vi "MGCC_FntStaMach_Flagtoevent.vi"(6 "ABN_recover":bool, 7 "Flags":bool[](array[boolean]), 8 "error in":errorcluster, 9 "M_OFF":bool, 10 "Pre_state":string, 11 "ABN_state":string="State1:OFF") -> (1 "error out":errorcluster, 2 "Event":bool[](array[boolean]), 3 "Previous_state":string)   [LabVIEW 2016]
doc: "-----------------------------------------------------------------------------------------------------------------------\nCopyright <2019> <The University of Tennessee at Knoxville and the University of Tennessee Research Foundation>\nThis software is released under BSD-3 \nhttps://opensource.org/licenses/BSD-3-Clause \nAdditional license options available at https://utrf.tennessee.edu/industry/sample-agreements/\n-----------------------------------------------------------------------------------------------------------------------"
uses:
  <vilib>/imath/engines/lvmath/Plug In/_Char/NIMS_CH_character datatype.ctl
  <vilib>/Utility/error.llb/Error Cluster From Error Code.vi
  Unplanned islanding/Sub Vis/UnplanISD_Global.vi
  <vilib>/imath/engines/lvmath/Plug In/_Char/NIMS_CH_String to Character Array.vi
  <vilib>/imath/engines/lvmath2/RunTimeEngine/IndexRead/NIMS V(S).vi
  <instcachedir>/0/NIMS V(S)_0488751826AF41519A22953C041130DC.lvgen/NIMS V(S)_0488751826AF41519A22953C041130DC_003.vi
  <vilib>/imath/engines/lvmath2/RunTimeEngine/ErrorHandling/NIMS_Create Error From Enums.vi
  <vilib>/imathl/engines/lvmath/Functions/Error Handling/Create Error.vi
  <vilib>/imath/engines/lvmath2/RunTimeSupport/NIMS_Compare Aggregates.vi
  <instcachedir>/0/NIMS_Compare Aggregates_FA3EBEB3749E48D38A57888B5ABBF163.lvgen/NIMS_Compare Aggregates_FA3EBEB3749E48D38A57888B5ABBF163_000.vi
  <vilib>/imath/engines/lvmath2/RunTimeEngine/NodeEndStatement/NIMS_NodeEndStatement_Output.vi
  <instcachedir>/0/NIMS_NodeEndStatement_Output_53EC0D466D134D7ABD903AC30B43404B.lvgen/NIMS_NodeEndStatement_Output_53EC0D466D134D7ABD903AC30B43404B_013.vi
  <vilib>/imath/engines/lvmath/Plug In/_Char/NIMS_CH_Character RV to String.vi
  <instcachedir>/0/NIMS_NodeEndStatement_Output_53EC0D466D134D7ABD903AC30B43404B.lvgen/NIMS_NodeEndStatement_Output_53EC0D466D134D7ABD903AC30B43404B_008.vi
  <vilib>/imath/engines/lvmath2/RunTimeEngine/ErrorHandling/NIMS_Finalize Error.vi
  <vilib>/ErrorRing/Error Ring.xnode
panel:
  out "error out 2":errorcluster
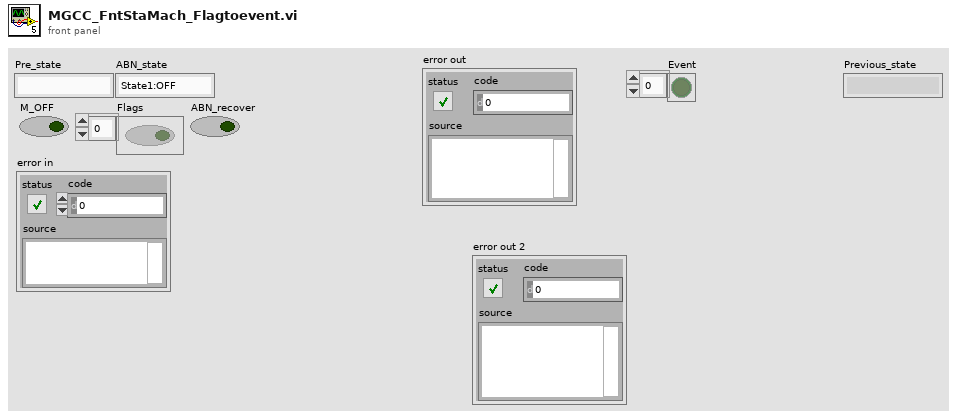
[diagram p1: front panel]
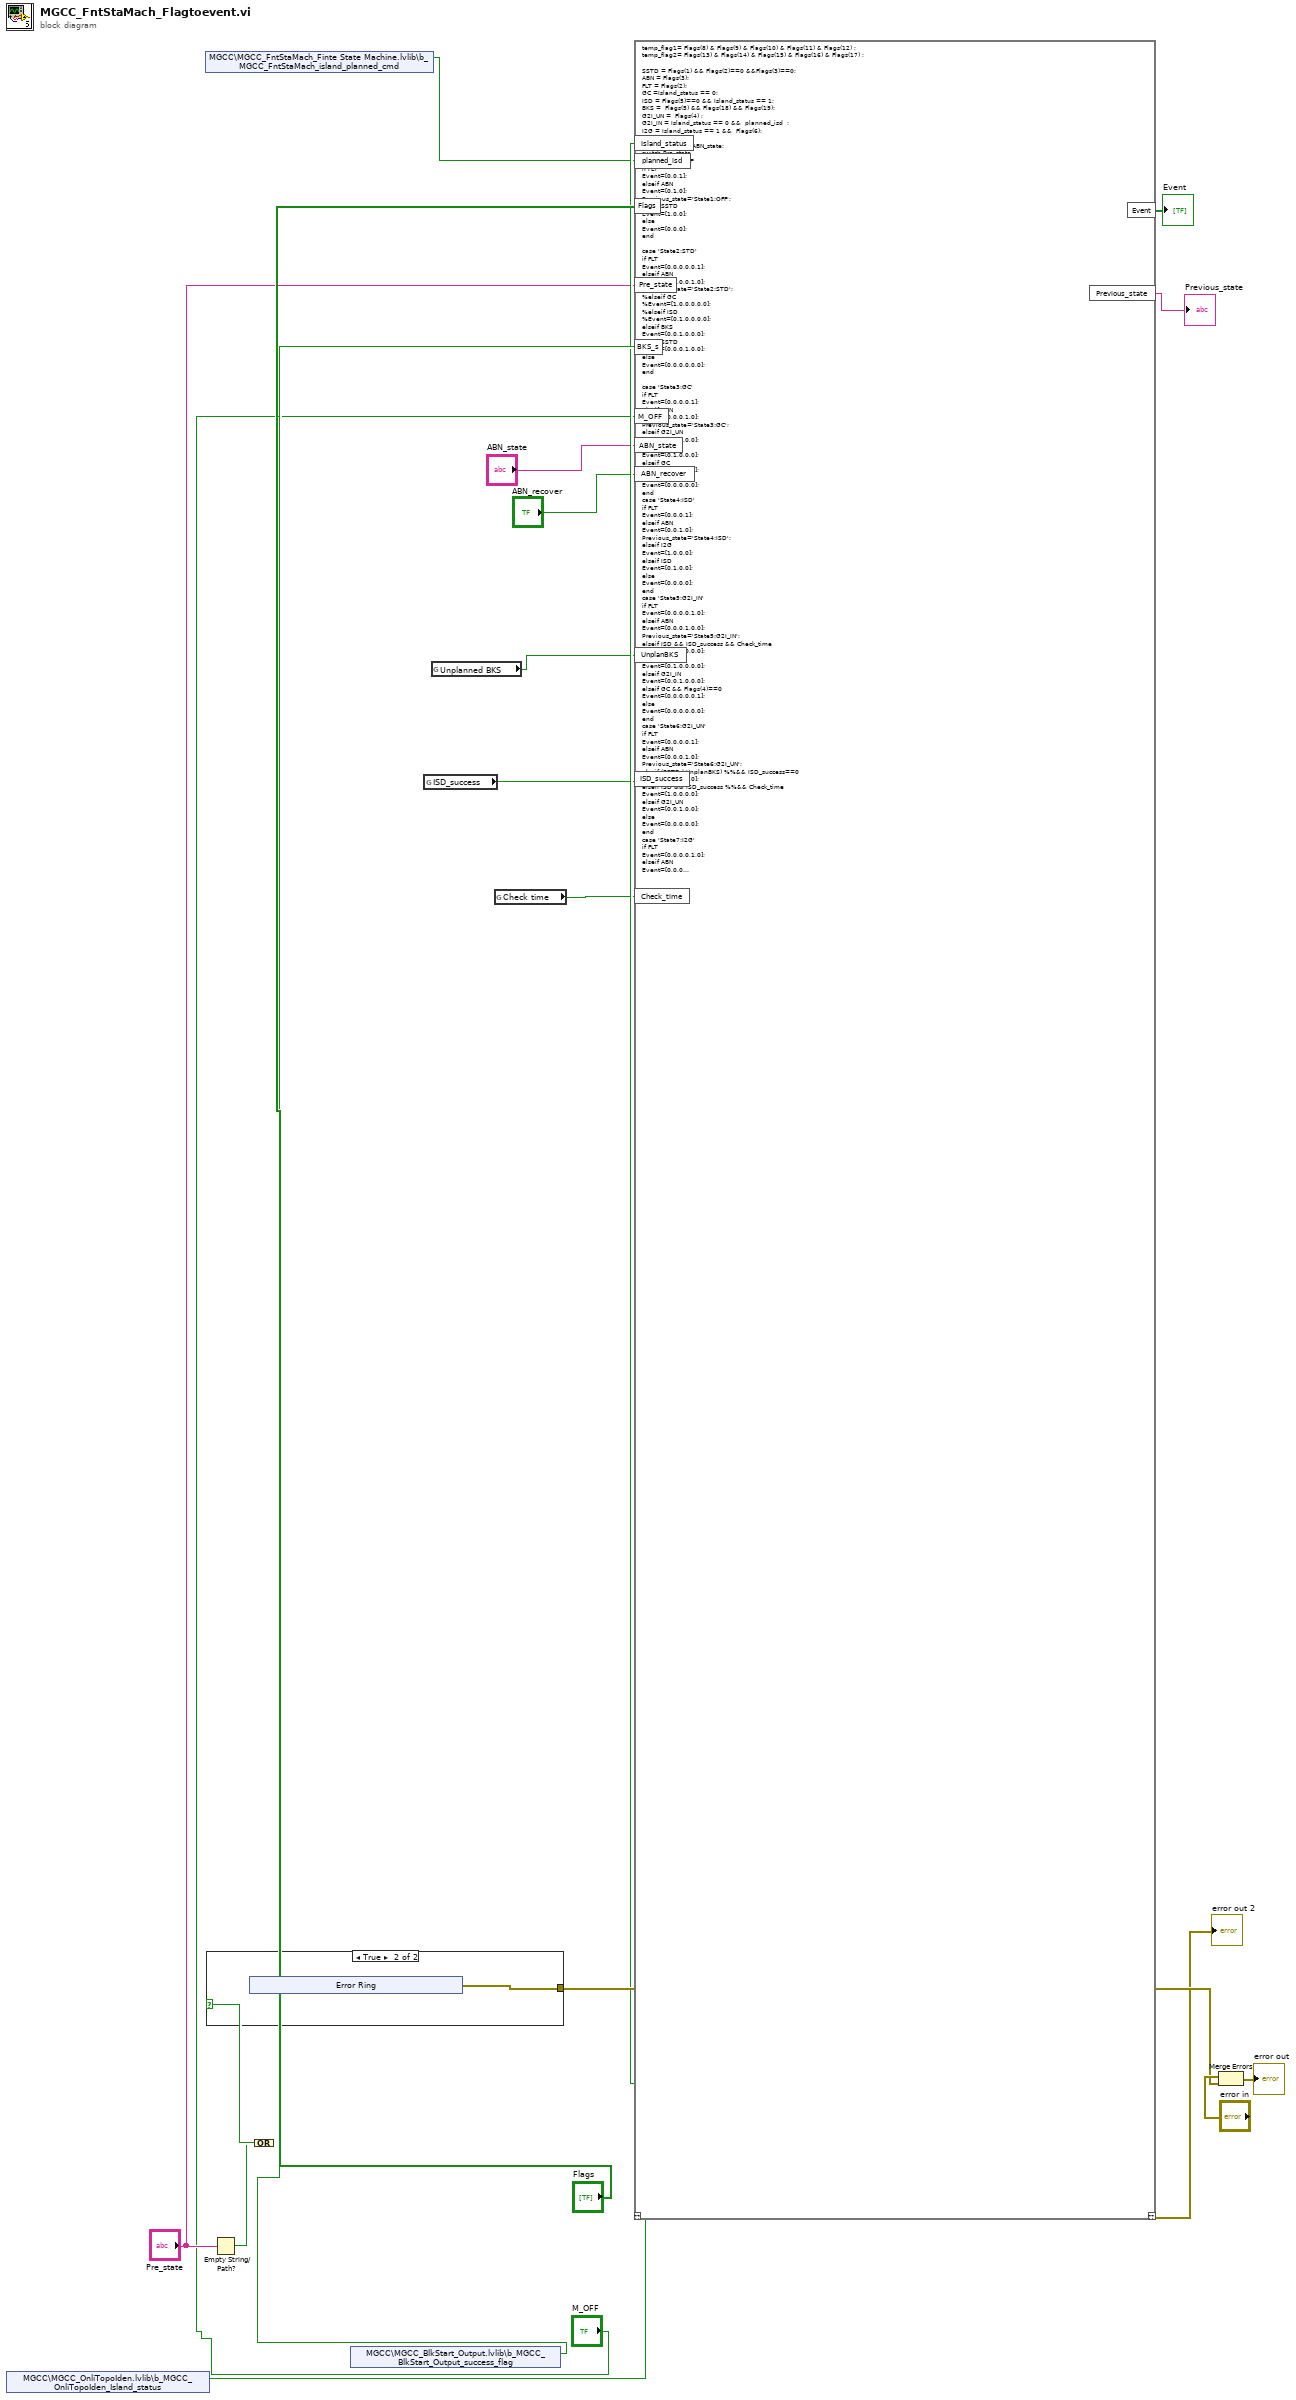
[diagram p0: block diagram]
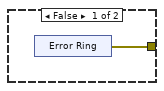
[diagram p2: hidden frame]
diagram:
  n1 = shared-variable "MGCC\\MGCC_OnliTopoIden.lvlib\\b_MGCC_OnliTopoIden_Island_status"() -> (w12:bool)  [unwired: 1 in, 1 out]
  n2 = shared-variable "MGCC\\MGCC_FntStaMach_Finte State Machine.lvlib\\b_MGCC_FntStaMach_island_planned_cmd"() -> (w5:bool)  [unwired: 1 in, 1 out]
  n3 = Empty String/Path?(string/path="Pre_state") -> (empty?=w13:bool)
  n4 = Compound Arithmetic op=OR(w13) -> (w15:bool)
  n5 = case shown="True" w15 {
    tunnel: [w20 w22] -> w14
    frame False {
      n6 = xnode "Error Ring"() -> ("error out"=w20:errorcluster)
    }
    frame True {
      n7 = xnode "Error Ring"() -> ("error out"=w22:errorcluster)
    }
  }
  n8 = shared-variable "MGCC\\MGCC_BlkStart_Output.lvlib\\b_MGCC_BlkStart_Output_success_flag"() -> (w18:bool)  [unwired: 1 in, 1 out]
  n9 = global read "UnplanISD_Global.vi" "ISD_success"() -> (w3:bool)
  n10 = global read "UnplanISD_Global.vi" "Unplanned BKS"() -> (w4:bool)
  n11 = global read "UnplanISD_Global.vi" "Check time"() -> (w2:bool)
  n12 = mathscript code="temp_flag1= Flags(8) & Flags(9) & Flags(10) & Flags(11) & Flags(12) ;\ntemp_flag2= Flags(13) & Flags(14) & Flags(15) & Flags(16) & Flags(17) ;\n\nSSTD = Flags(1) && Flags(2)==0 &&Flags(3)==0;\nABN = Flags(3);\nFLT = Flags(2);\nGC =Island_status == 0;\nISD = Flags(5)==0 && Island_status == 1;\nBKS =  Flags(5) && Flags(18) && Flags(19);\nG2I_UN =  Flags(4) ;\nG2I_IN = Island_status == 0 &&  planned_isd  ;\nI2G = Island_status == 1 &&  Flags(6);\nOFF = M_OFF;\nPrevious_state=ABN_state;\nswitch Pre_state\ncase 'State1:OFF'\nif FLT\nEvent=[0,0,1];\nelseif ABN\nEvent=[0,1,0];\nPrevious_state='State1:OFF';\nelseif SSTD\nEvent=[1,0,0];\nelse\nEvent=[0,0,0];\nend \n\ncase 'State2:STD'\nif FLT\nEvent=[0,0,0,0,0,1];\nelseif ABN\nEvent=[0,0,0,0,1,0];\nPrevious_state='State2:STD';\n%elseif GC\n%Event=[1,0,0,0,0,0];\n%elseif ISD\n%Event=[0,1,0,0,0,0];\nelseif BKS\nEvent=[0,0,1,0,0,0];\nelseif SSTD\nEvent=[0,0,0,1,0,0];\nelse\nEvent=[0,0,0,0,0,0];\nend \n\ncase 'State3:GC'\nif FLT\nEvent=[0,0,0,0,1];\nelseif ABN\nEvent=[0,0,0,1,0];\nPrevious_state='State3:GC';\nelseif G2I_UN\nEvent=[1,0,0,0,0];\nelseif G2I_IN\nEvent=[0,1,0,0,0];\nelseif GC\nEvent=[0,0,1,0,0];\nelse\nEvent=[0,0,0,0,0];\nend\ncase 'State4:ISD'\nif FLT\nEvent=[0,0,0,1];\nelseif ABN\nEvent=[0,0,1,0];\nPrevious_state='State4:ISD';\nelseif I2G\nEvent=[1,0,0,0];\nelseif ISD\nEvent=[0,1,0,0];\nelse\nEvent=[0,0,0,0];\nend\ncase 'State5:G2I_IN'\nif FLT\nEvent=[0,0,0,0,1,0];\nelseif ABN\nEvent=[0,0,0,1,0,0];\nPrevious_state='State5:G2I_IN';\nelseif ISD && ISD_success && Check_time\nEvent=[1,0,0,0,0,0];\nelseif SSTD\nEvent=[0,1,0,0,0,0];\nelseif G2I_IN\nEvent=[0,0,1,0,0,0];\nelseif GC && Flags(4)==0 \nEvent=[0,0,0,0,0,1];\nelse\nEvent=[0,0,0,0,0,0];\nend\ncase 'State6:G2I_UN'\nif FLT\nEvent=[0,0,0,0,1];\nelseif ABN\nEvent=[0,0,0,1,0];\nPrevious_state='State6:G2I_UN';\nelseif (SSTD | UnplanBKS) %%&& ISD_success==0\nEvent=[0,1,0,0,0];\nelseif ISD && ISD_success %%&& Check_time\nEvent=[1,0,0,0,0];\nelseif G2I_UN\nEvent=[0,0,1,0,0];\nelse\nEvent=[0,0,0,0,0];\nend\ncase 'State7:I2G'\nif FLT\nEvent=[0,0,0,0,1,0];\nelseif ABN\nEvent=[0,0,0,1,0,0];\nPrevious_state='State7:I2G';\nelseif GC\nEvent=[1,0,0,0,0,0];\nelseif SSTD\nEvent=[0,1,0,0,0,0];\nelseif I2G\nEvent=[0,0,1,0,0,0];\nelseif ISD && Flags(6) ==0\nEvent=[0,0,0,0,0,1];\nelse\nEvent=[0,0,0,0,0,0];\nend\ncase 'State8:BKS'\nif FLT\nEvent=[0,0,0,0,1];\nelseif ABN\nEvent=[0,0,0,1,0];\nPrevious_state='State8:BKS';\nelseif ISD && BKS_s\nEvent=[1,0,0,0,0];\nelseif SSTD\nEvent=[0,1,0,0,0];\nelseif BKS\nEvent=[0,0,1,0,0];\nelse\nEvent=[0,0,0,0,0];\nend\ncase 'State9:ABN'\nif FLT\nEvent=[0,0,0,0,0,0,0,0,1];\nelseif ABN\nEvent=[0,0,0,0,0,0,0,1,0];\nelse\nswitch ABN_state\ncase 'State2:STD'\nEvent=[1,0,0,0,0,0,0,0,0];\ncase 'State3:GC'\nEvent=[0,1,0,0,0,0,0,0,0];\ncase 'State4:ISD'\nEvent=[0,0,1,0,0,0,0,0,0];\ncase 'State6:G2I_UN'\nEvent=[0,0,0,0,1,0,0,0,0];\ncase 'State5:G2I_IN'\nEvent=[0,0,0,1,0,0,0,0,0];\ncase 'State7:I2G'\nEvent=[0,0,0,0,0,1,0,0,0];\ncase 'State8:BKS'\nEvent=[0,0,0,0,0,0,1,0,0];\notherwise\nEvent=[0,0,0,0,0,0,0,1,0];\nend\nend\n\ncase 'State10:FLT'\nif FLT\nEvent=[1,0,0,0];\nelseif ABN\nEvent=[0,1,0,0];\nelseif SSTD\nEvent=[0,0,1,0];\nelseif OFF\nEvent=[0,0,0,1];\nelse\nEvent=[0,0,0,0];\nend\notherwise\nEvent=[0,0,0,0,0,0,0,1,0];\nend"("Flags"="Flags", "Pre_state"="Pre_state", "M_OFF"="M_OFF", "BKS_s"=w18, "Island_status"=w12, "ABN_state"="ABN_state", "ABN_recover"="ABN_recover", "planned_isd"=w5, "UnplanBKS"=w4, "ISD_success"=w3, "Check_time"=w2) -> ("??"=→"error out 2":errorcluster, "Event"=→"Event":bool[], "Previous_state"=→"Previous_state":string)  [unwired: 1 in]
  n13 = Merge Errors("error in", w14) -> (→"error out":errorcluster)
